vi "gyro -- sourcer async.vi"(11 "sourcer event pair":T1) -> ()   [LabVIEW 2018]
uses:
  server talk-to-back pair.ctl
  server talkback message type.ctl
  server talkto message type.ctl
  mfli reader event.ctl
  MFLI frontend action.ctl
  publisher action.ctl
  data source action.ctl
  PLL data source.ctl
panel:
  in  "all":enum32{"all", "all 2"}(tab)
  out "read Voltage (V)":cdb=2.0706635468928775e-07+4.4716444398634134e-07i format="%#10_10f"
  in  "read status":bool
  out "read Voltage X (V)":dbl=2.0706635468928775e-07 format="%#11_11f"
  out "read Voltage Y (V)":dbl=4.4716444398634134e-07 format="%#11_11f"
  in  "delay-read (msec)":i64=20
  out "zi freq (Hz)":dbl=99999.99999990905 format="%-#.3f"
  in  "MFLI Address":string="dev4307"
  in  "amplitude (V)":dbl=0.01
  in  "set amp! :m":bool
  in  "start  !":bool
  in  "stop  !":bool
  out "Stopped?":bool
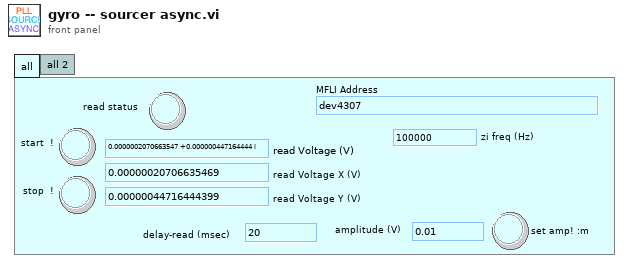
[diagram p1: front panel]
types:
  T1 = typedef "server talk-to-back pair.ctl" = cluster{"talkback event":refnum<user-event>, "talkto event":refnum<user-event>}
  T2 = typedef "server talkto message type.ctl" = cluster{"message":enum16{"stop", "start", "update pars", "update request", "new", "launch", "exit", "get", "reset", "pause", "unpause"}}
  T3 = typedef "MFLI frontend action.ctl" = enum16{"read", "writeread", "open", "close", "write"}
  T4 = typedef "mfli reader event.ctl" = enum16{"start", "stop", "exit"}
  T5 = typedef "publisher action.ctl" = enum16{"set", "get", "init", "check"}
  T6 = typedef "PLL data source.ctl" = enum16{"meta", "MFLI", "SRS865A"}
  T7 = typedef "data source action.ctl" = enum16{"set", "get", "init", "set-and-get", "init source"}
  T8 = typedef "Zurich Instruments LabOne.lvlib/ziTypeHandle.ctl" = cluster{"handleValid":bool, "Conn":u64, "Path Prefix":string, "Handle":u64, "Connected":bool, "Clockbase(s)":dbl}
  T9 = enum16{"stop", "start", "update pars", "update request", "new", "launch", "exit", "get", "reset", "pause", "unpause"}
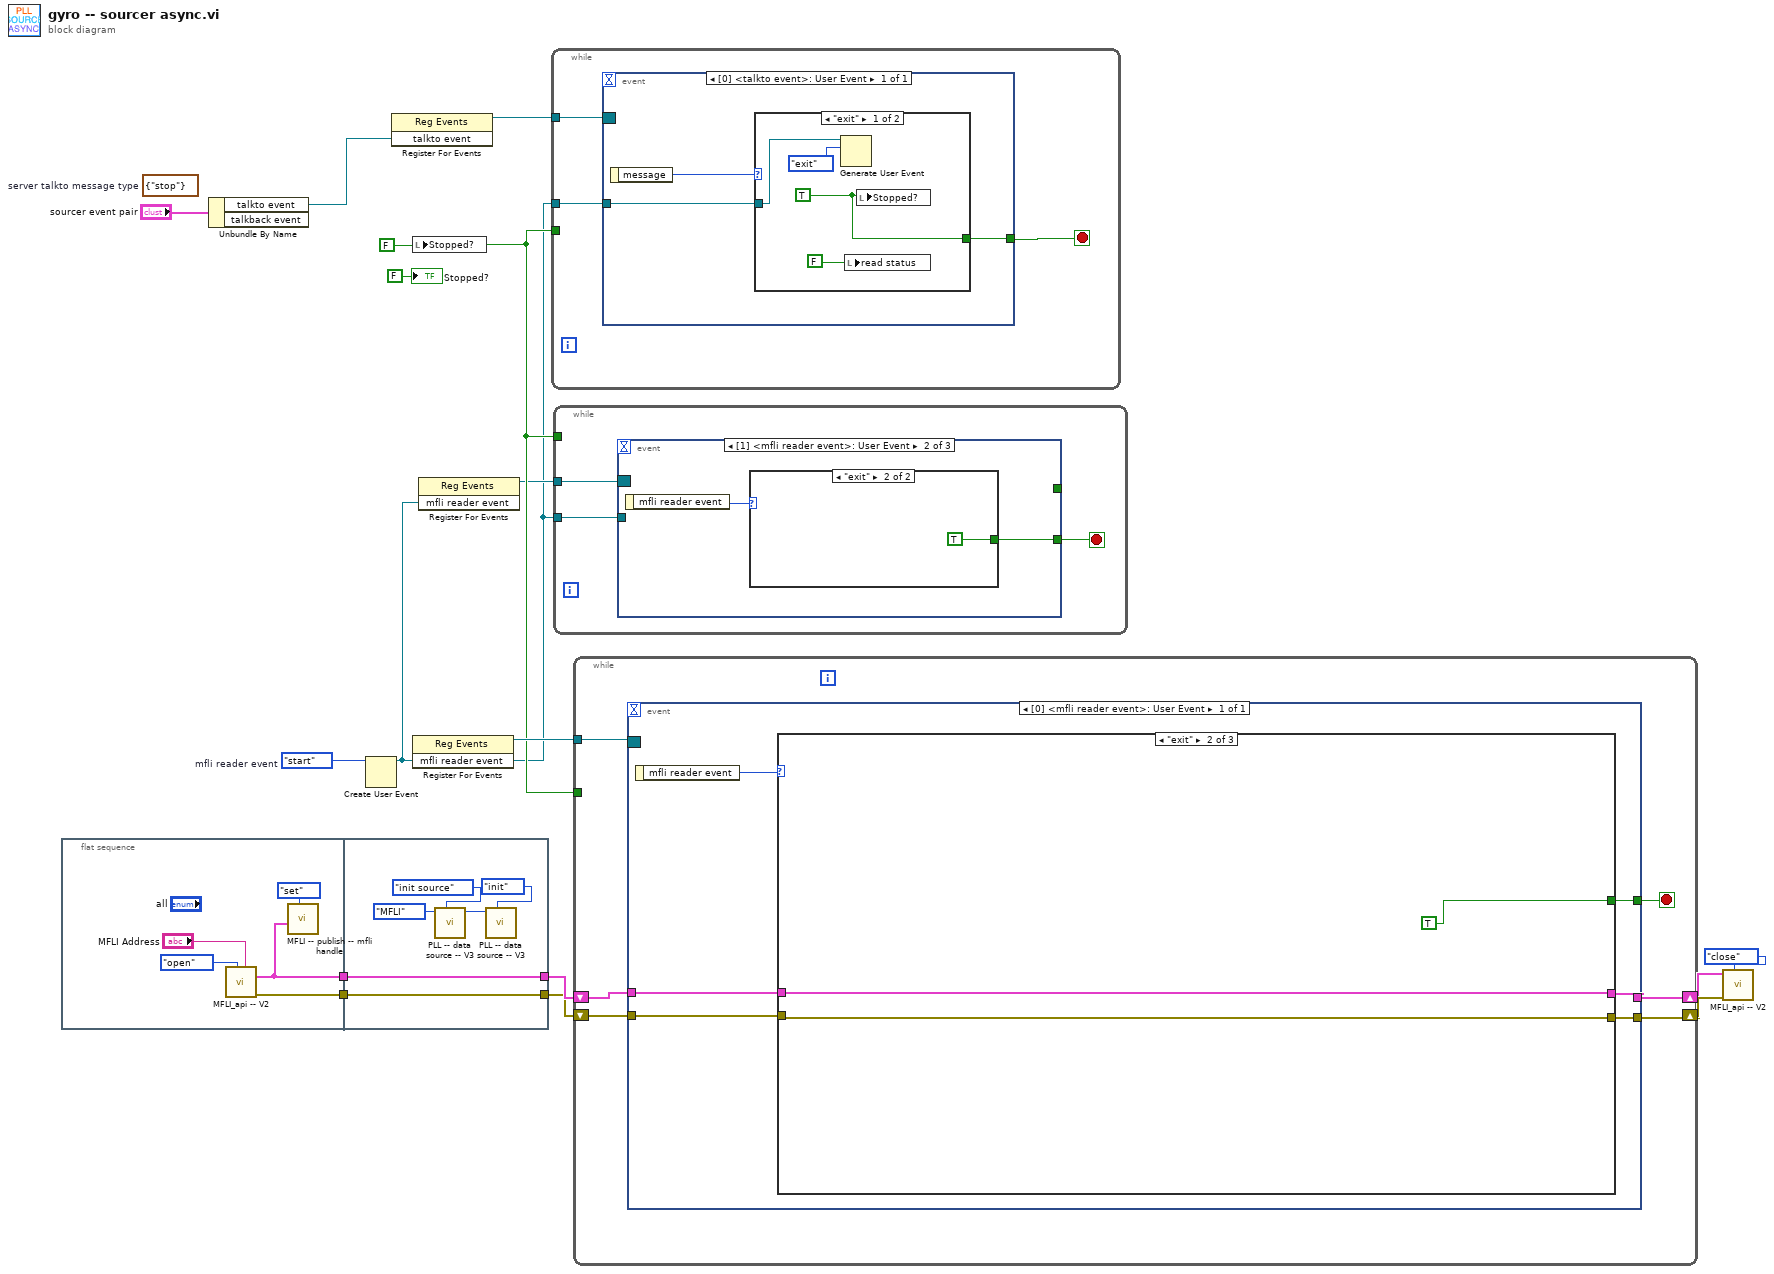
[diagram p0: block diagram]
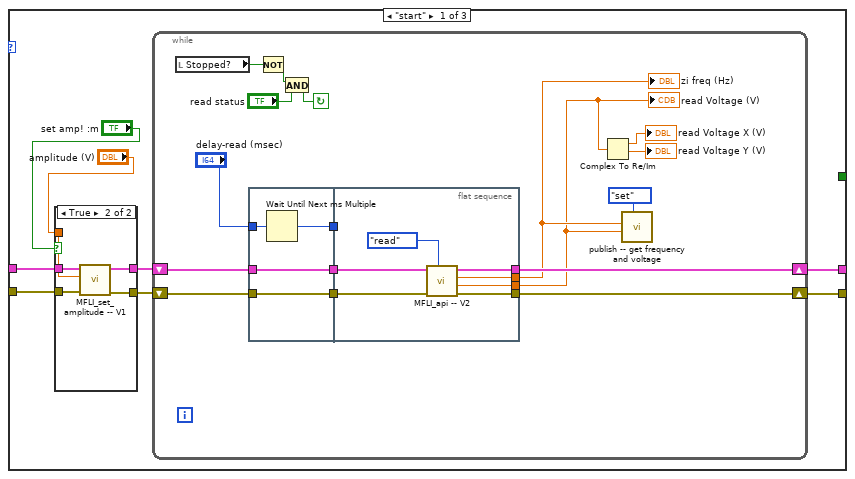
[diagram p3: hidden frame]
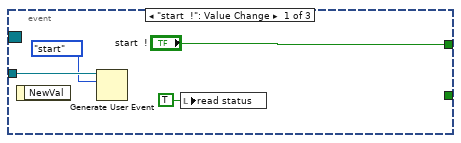
[diagram p6: hidden frame]
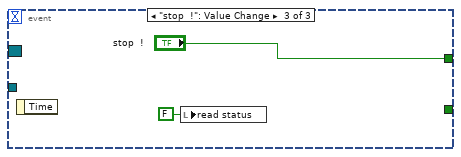
[diagram p8: hidden frame]
diagram:
  (unwired) T2 {"message"=enum."stop"}  # server talkto message type
  w3 = FALSE ("Stop")
  w15 = mfli_reader_event."start"  # mfli reader event
  n1 = flat-sequence {
    tunnel: [w18] -> w5
    tunnel: [w17] -> w4
    tunnel: [w26] -> w10
    tunnel: [w27] -> w11
    tunnel: w5 -> [w27]
    tunnel: w4 -> [w26]
    frame #0 {
      n2 = call "MFLI_api -- V2.vi"("MFLI Address"="MFLI Address", "MFLI frontend action"=MFLI_frontend_action."open") -> ("Error Out"=w17:errorcluster, "Handle Out"=w18:T8)  [unwired: 6 in, 2 out]
      n3 = call "MFLI -- publish -- mfli handle.vi"("publisher action"=publisher_action."set", "Handle IN"=w18) -> ()  [unwired: 9 in, 1 out]
    }
    frame #1 {
      n4 = call "PLL -- data source -- V3.vi"("data source action"=data_source_action."init source", "PLL data source"=PLL_data_source."MFLI") -> ("PLL data source OUT"=w25:T6)  [unwired: 7 in, 2 out]
      n5 = call "PLL -- data source -- V3.vi"("data source action"=data_source_action."init", "PLL data source"=w25) -> ()  [unwired: 7 in, 3 out]
    }
  }
  n6 = Unbundle By Name("sourcer event pair") -> ("talkto event"=w7:refnum<user-event>)  [unwired: 1 out]
  n7 = Create User Event(user event datatype=w15) -> (user event=w1:refnum<user-event>)  [unwired: 1 in, 1 out]
  n8 = register-events(w7) -> (reference out=w9:refnum<event-registration>)  [unwired: 2 in, 1 out]
  n9 = local write "Stopped?"(w3) -> ()
  n10 = register-events(w1) -> (reference out=w16:refnum<event-registration>)  [unwired: 2 in, 1 out]
  n11 = register-events(w1) -> (reference out=w2:refnum<event-registration>)  [unwired: 2 in, 1 out]
  n12 = while {
    tunnel: w9 -> [w30]
    tunnel: w3 -> [_]
    tunnel: w1 -> [w28]
    stop <- w29 stop-if-true
    n13 = event shown="[0] <talkto event>: User Event" {
      selector: w30 -> [_]
      dyn-events: _ -> [_]
      timeout: _ -> [_]
      tunnel: [w32] -> w29
      tunnel: w28 -> [w31]
      event User Event {
        n14 = event-data() -> ("message"=w33:T9)  [unwired: 1 in]
        n15 = case shown="\"exit\"" w33 {
          tunnel: [w36 _] -> w32
          tunnel: w31 -> [w35 _]
          frame "exit" {
            w36 = TRUE ("Stoped?")
            n16 = Generate User Event(user event=w35, event data cluster=mfli_reader_event."exit" ("event data")) -> ()  [unwired: 2 in, 2 out]
            n17 = local write "read status"(FALSE ("read status")) -> ()
            n18 = local write "Stopped?"(w36) -> ()
          }
          frame "get", Default {
          }
        }
      }
    }
  }
  n19 = while {
    tunnel: w1 -> [w40]
    tunnel: w3 -> [_]
    tunnel: w2 -> [w39]
    stop <- w38 stop-if-true
    n20 = event shown="[1] <mfli reader event>: User Event" {
      selector: w39 -> [_ _ _]
      dyn-events: _ -> [_ _ _]
      timeout: _ -> [_ _ _]
      tunnel: ["start  !" _ "stop  !"] -> _
      tunnel: w40 -> [w42 _ _]
      tunnel: [_ w45 _] -> w38
      event "start  !": Value Change {
        n21 = event-data() -> ()  [unwired: 1 in, 1 out]
        n22 = Generate User Event(user event=w42, event data cluster=mfli_reader_event."start" ("event data")) -> ()  [unwired: 2 in, 2 out]
        n23 = local write "read status"(TRUE ("read status")) -> ()
      }
      event User Event {
        n24 = event-data() -> ("mfli reader event"=w46:T4)  [unwired: 1 in]
        n25 = case shown="\"exit\"" w46 {
          tunnel: [_ TRUE] -> w45
          frame "start", Default {
          }
          frame "exit" {
          }
        }
      }
      event "stop  !": Value Change {
        n26 = event-data() -> ()  [unwired: 1 in, 1 out]
        n27 = local write "read status"(FALSE ("read status")) -> ()
      }
    }
  }
  n28 = while {
    tunnel: w16 -> [w55]
    shift-right: [w53] -> w12
    shift-left: w11 -> [w52]
    shift-right: [w54] -> w13
    shift-left: w10 -> [w51]
    tunnel: w3 -> [_]
    stop <- w50 stop-if-true
    n29 = event shown="[0] <mfli reader event>: User Event" {
      selector: w55 -> [_]
      dyn-events: _ -> [_]
      timeout: _ -> [_]
      tunnel: w52 -> [w61]
      tunnel: w51 -> [w60]
      tunnel: [w59] -> w54
      tunnel: [w58] -> w53
      tunnel: [w56] -> w50
      event User Event {
        n30 = event-data() -> ("mfli reader event"=w57:T4)  [unwired: 1 in]
        n31 = case shown="\"exit\"" w57 {
          tunnel: w61 -> [w68 w107 w109]
          tunnel: w60 -> [w66 w106 w108]
          tunnel: [w63 w106 w108] -> w59
          tunnel: [w62 w107 w109] -> w58
          tunnel: [_ TRUE _] -> w56
          frame "start" {
            n32 = case shown="True" "set amp! :m" {
              tunnel: w68 -> [w71 w76]
              tunnel: [w71 w75] -> w67
              tunnel: w66 -> [w70 w74]
              tunnel: [w70 w73] -> w65
              tunnel: "amplitude (V)" -> [_ w72]
              frame False {
              }
              frame True {
                n33 = call "MFLI_set_amplitude -- V1.vi"("Error In"=w74, "Amp in (V)"=w72, "Handle In"=w76) -> ("Error Out"=w73:errorcluster, "Handle Out"=w75:T8)  [unwired: 5 in, 2 out]
              }
            }
            n34 = while {
              shift-right: [w92] -> w63
              shift-left: w65 -> [w93]
              shift-right: [w90] -> w62
              shift-left: w67 -> [w91]
              stop <- w79 continue-if-true
              n35 = local read "Stopped?"() -> (w77:bool)
              n36 = flat-sequence {
                tunnel: [w97] -> w89
                tunnel: "delay-read (msec)" -> [w96]
                tunnel: [w95] -> w88
                tunnel: w93 -> [w95]
                tunnel: w91 -> [w94]
                tunnel: [w94] -> w87
                tunnel: w89 -> [_]
                tunnel: [w102] -> w81
                tunnel: [w101] -> w82
                tunnel: w88 -> [w104]
                tunnel: [w103] -> w92
                tunnel: w87 -> [w100]
                tunnel: [w99] -> w90
                frame #0 {
                  n37 = Wait Until Next ms Multiple(millisecond multiple=w96) -> (millisecond timer value=w97:u32)
                }
                frame #1 {
                  n38 = call "MFLI_api -- V2.vi"("MFLI frontend action"=MFLI_frontend_action."read", "Error In"=w104, "Handle In"=w100) -> ("Error Out"=w103:errorcluster, "z out (V)"=w102:cdb, "Freq out (Hz)"=w101:dbl, "Handle Out"=w99:T8)  [unwired: 5 in]
                }
              }
              n39 = Not(x=w77) -> (.not. x?=w80:bool)
              n40 = And(x=w80, y="read status") -> (x .and. y?=w79:bool)
              n41 = Complex To Re/Im(x + iy=w81) -> (x=→"read Voltage X (V)":dbl, y=→"read Voltage Y (V)":dbl)
              n42 = call "publish -- get frequency and voltage.vi"("publisher action"=publisher_action."set", "Voltage IN (V)"=w81, "freq IN (Hz)"=w82) -> ()  [unwired: 6 in, 3 out]
              "read Voltage (V)" <- w81
              "zi freq (Hz)" <- w82
            }
          }
          frame "exit" {
          }
          frame "stop", Default {
          }
        }
      }
    }
  }
  n43 = call "MFLI_api -- V2.vi"("MFLI frontend action"=MFLI_frontend_action."close", "Error In"=w13, "Handle In"=w12) -> ()  [unwired: 5 in, 4 out]
  "Stopped?" <- FALSE ("Stoped?")
